vi "Solve1.vi"(8 "Error In":errorcluster, 11 "object in":refnum<class "2025_2.lvclass">) -> (0 "Error Out":errorcluster, 2 "Result":u64, 3 "object out":refnum<class "2025_2.lvclass">)   [LabVIEW 2025, in "2025_2.lvclass"]
uses:
  2025_2.lvclass
  2025_2.lvclass/2025_2.ctl
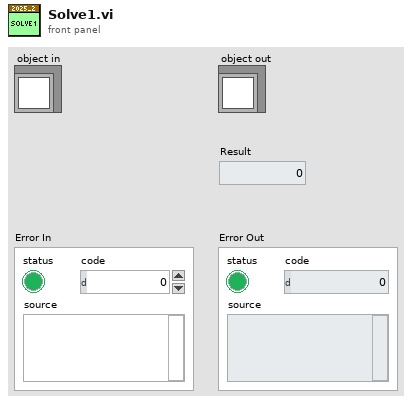
[diagram p1: front panel]
types:
  T1 = typedef "2025_2.lvclass/Range.ctl" = cluster{"Start":u64, "End":u64}
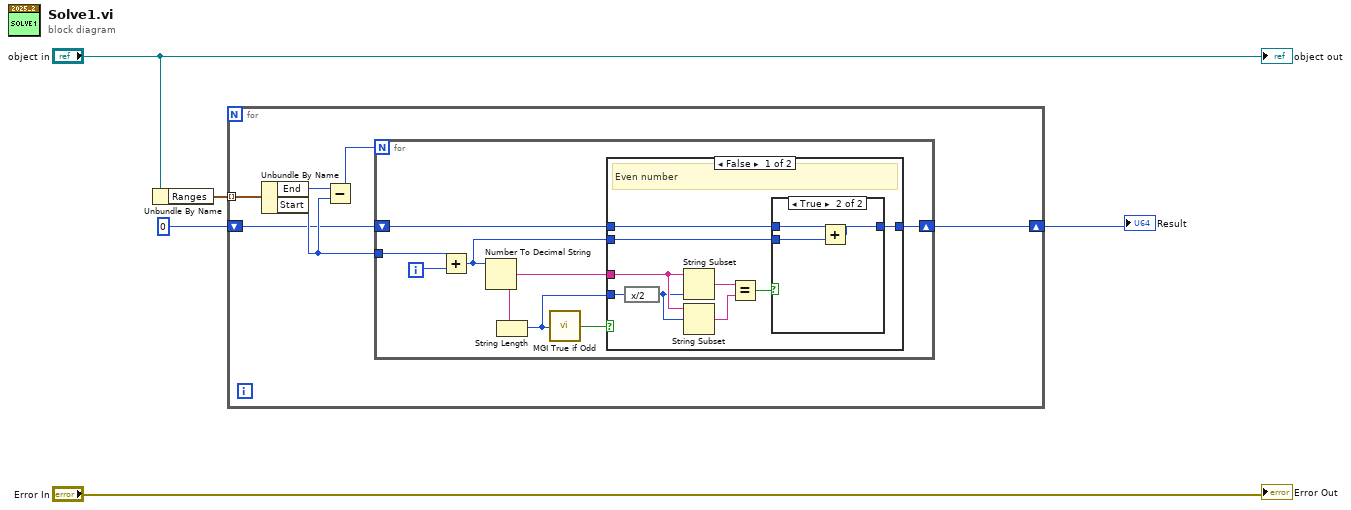
[diagram p0: block diagram]
diagram:
  n1 = Unbundle By Name("object in") -> ("Ranges"=w3:T1[])
  n2 = for {
    tunnel: w3 -> [w11] mode=indexing
    shift-right: [w7] -> w2
    shift-left: u64 0 -> [w6]
    n3 = Unbundle By Name(w11) -> ("End"=w10:u64, "Start"=w8:u64)
    n4 = Subtract(x=w10, y=w8) -> (x-y=w9:u64)
    n5 = for {
      N: w9 -> [_]
      tunnel: w8 -> [w19]
      shift-right: [w12] -> w7
      shift-left: w6 -> [w14]
      i -> [w18]
      n6 = Add(x=w19, y=w18) -> (x+y=w13:u64)
      n7 = Number To Decimal String(number=w13) -> (decimal integer string=w16:string)  [unwired: 1 in]
      n8 = String Length(string=w16) -> (length=w15:i32)
      n9 = call <userlib>:"MGI True if Odd.vi"("Integer"=w15) -> ("Odd?"=w17:bool)
      n10 = case shown="False" w17 {
        tunnel: w16 -> [w27 _]
        tunnel: w15 -> [w28 _]
        tunnel: w14 -> [w22 w33]
        tunnel: w13 -> [w21 _]
        tunnel: [w20 w33] -> w12
        frame False {
          # "Even number"
          n11 = expression code="x/2"(w28) -> (w26:i32)
          n12 = String Subset(string=w27, length (rest)=w26) -> (substring=w25:string)  [unwired: 1 in]
          n13 = String Subset(string=w27, offset (0)=w26) -> (substring=w24:string)  [unwired: 1 in]
          n14 = Equal?(x=w25, y=w24) -> (x = y?=w23:bool)
          n15 = case shown="True" w23 {
            tunnel: w22 -> [w29 w32]
            tunnel: w21 -> [_ w31]
            tunnel: [w29 w30] -> w20
            frame False {
            }
            frame True {
              n16 = Add(x=w32, y=w31) -> (x+y=w30:u64)
            }
          }
        }
        frame True {
          # "Odd number ignore"
        }
      }
    }
  }
  "Result" <- w2
  "Error Out" <- "Error In"
  "object out" <- "object in"
